vi "Database Recordset Get Fields Count.vi"(8 "error in (no error)":errorcluster caption="错误输入（无错误）", 11 "Database Recordset 输入":refnum<class "Database Recordset.lvclass"> caption="DNL_LabVIEW Object in") -> (0 "error out":errorcluster caption="错误输出", 2 "Count":i32, 3 "Database Recordset 输出":refnum<class "Database Recordset.lvclass"> caption="DNL_LabVIEW Object out")   [LabVIEW 2011, in "Database Recordset.lvclass"]
uses:
  Database Recordset.lvclass
  Database Recordset.lvclass/Database Recordset.ctl
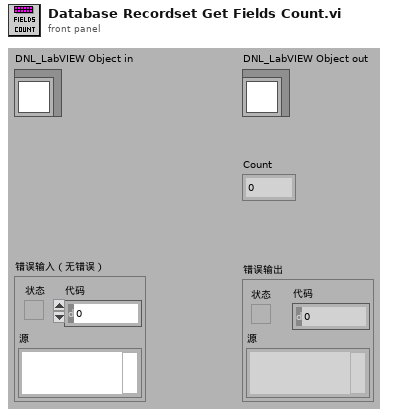
[diagram p1: front panel]
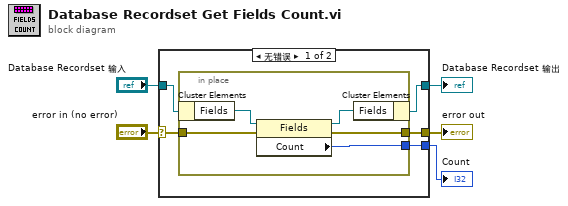
[diagram p0: block diagram]
diagram:
  n1 = case shown="无错误" "error in (no error)" {
    selector: "error in (no error)" -> [w10 w17]
    tunnel: [w9 w17] -> w4
    tunnel: [w6 w16] -> w2
    tunnel: "Database Recordset 输入" -> [w7 w16]
    tunnel: [w8 _] -> w1
    frame No Error {
      n2 = in-place {
        in-place-border: w10 -> [w15]
        in-place-border: [w14] -> w9
        in-place-border: [w13] -> w8
        n3 = in-place-cluster #1(w7) -> ("Fields"=w12:refnum<k7>)
        n4 = property class="Fields"(reference=w12, error in=w15) -> (reference out=w11:refnum<k7>, error out=w14:errorcluster, "Count"=w13:i32)
        n5 = in-place-cluster #1("Fields"=w11) -> (w6:refnum<class "Database Recordset.lvclass">)
      }
    }
    frame Error {
    }
  }
  "error out" <- w4
  "Database Recordset 输出" <- w2
  "Count" <- w1
